vi "Storage Command Handler Test.vi"(11 "Buttons":bool[](array[boolean])) -> ()   [LabVIEW 2019]
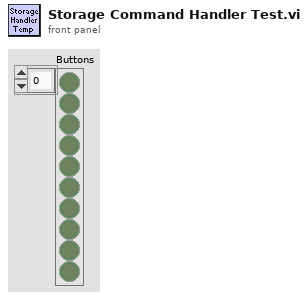
[diagram p1: front panel]
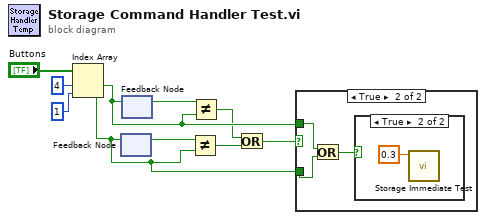
[diagram p0: block diagram]
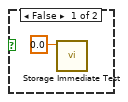
[diagram p3: hidden frame]
diagram:
  n1 = Index Array(array="Buttons", index #1=4 ("index"), index #2=1 ("index")) -> (element #1=w7:bool, element #2=w6:bool)
  n2 = feedback #1() -> (w3:bool)  [unwired: 1 in]
  n3 = feedback-in #1(w6) -> ()
  n4 = feedback #2() -> (w5:bool)  [unwired: 1 in]
  n5 = feedback-in #2(w7) -> ()
  n6 = Not Equal?(x=w3, y=w6) -> (x != y?=w2:bool)
  n7 = Not Equal?(x=w5, y=w7) -> (x != y?=w1:bool)
  n8 = Or(x=w1, y=w2) -> (x .or. y?=w4:bool)
  n9 = case shown="True" w4 {
    tunnel: w6 -> [_ w12]
    tunnel: w7 -> [_ w11]
    frame False {
    }
    frame True {
      n10 = Or(x=w11, y=w12) -> (x .or. y?=w13:bool)
      n11 = case shown="True" w13 {
        frame False {
          n12 = call "Storage Immediate Test.vi"("Setpoint"=0.0) -> ()  [unwired: 10 in, 1 out]
        }
        frame True {
          n13 = call "Storage Immediate Test.vi"("Setpoint"=0.3) -> ()  [unwired: 10 in, 1 out]
        }
      }
    }
  }
